vi "Nanonisframe.vi"(0 "x":dbl, 1 "z":dbl) -> (8 "X Out":dbl, 10 "Z Out":dbl, 11 "Target X":dbl, 12 "Speed":dbl, 13 "Target Z":dbl, 14 "FO X":dbl, 15 "FO Z":dbl, 16 "FW":dbl, 17 "FH":dbl)   [LabVIEW 2017]
uses:
  <userlib>/Nanonis Prog Interface V5/Nanonis Prog Interface.lvlib
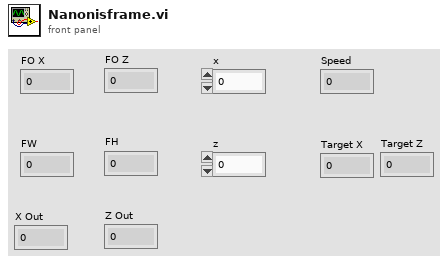
[diagram p1: front panel]
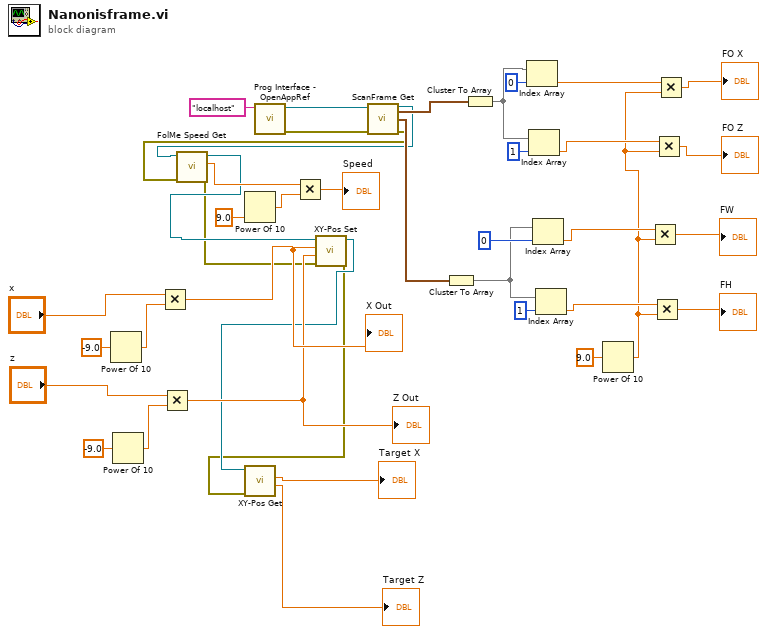
[diagram p0: block diagram]
diagram:
  n1 = Power Of 10(x=-9.0) -> (10^x=w16:dbl)
  n2 = Power Of 10(x=-9.0) -> (10^x=w13:dbl)
  n3 = Multiply(x="x", y=w16) -> (x*y=w9:dbl)
  "X Out" <- w9
  n4 = Multiply(x="z", y=w13) -> (x*y=w8:dbl)
  "Z Out" <- w8
  n5 = Power Of 10(x=9.0) -> (10^x=w19:dbl)
  n6 = call <userlib>:"Prog Interface - OpenAppRef.vi"("Machine name (local machine IP)"="localhost") -> ("Error out"=w4:errorcluster, "Application reference"=w40:refnum<vi>)  [unwired: 5 in]
  n7 = call <userlib>:"ScanFrame Get.vi"("Application ref in"=w40, "error in (no error)"=w4) -> ("Application ref out"=w21:refnum<vi>, "Center coordinates (m)"=w39:cluster{"Xc":sgl, "Yc":sgl}, "Size (m)"=w35:cluster{"Width":sgl, "Height":sgl}, "error out"=w3:errorcluster)  [unwired: 9 in, 1 out]
  n8 = call <userlib>:"FolMe Speed Get.vi"("error in (no error)"=w3, "Application ref in"=w21) -> ("error out"=w2:errorcluster, "Speed (m/s)"=w18:sgl, "Application ref out"=w10:refnum<vi>)  [unwired: 4 in, 1 out]
  n9 = Multiply(x=w18, y=w19) -> (x*y=→"Speed":dbl)
  n10 = call <userlib>:"XY-Pos Set.vi"("error in (no error)"=w2, "Y (m)"=w8, "X (m)"=w9, "Application ref in"=w10) -> ("error out"=w1:errorcluster, "Application ref out"=w7:refnum<vi>)  [unwired: 4 in]
  n11 = call <userlib>:"XY-Pos Get.vi"("error in (no error)"=w1, "Application ref in"=w7) -> ("Y (m)"=→"Target Z":sgl, "X (m)"=→"Target X":sgl)  [unwired: 5 in, 2 out]
  n12 = Cluster To Array(cluster=w35) -> (array=w32:sgl[])
  n13 = Cluster To Array(cluster=w39) -> (array=w38:sgl[])
  n14 = Index Array(array=w38, index=0) -> (element=w31:sgl)
  n15 = Index Array(array=w38, index=1) -> (element=w30:sgl)
  n16 = Index Array(array=w32, index=0) -> (element=w29:sgl)
  n17 = Index Array(array=w32, index=1) -> (element=w28:sgl)
  n18 = Power Of 10(x=9.0) -> (10^x=w26:dbl)
  n19 = Multiply(x=w29, y=w26) -> (x*y=→"FW":dbl)
  n20 = Multiply(x=w28, y=w26) -> (x*y=→"FH":dbl)
  n21 = Multiply(x=w30, y=w26) -> (x*y=→"FO Z":dbl)
  n22 = Multiply(x=w31, y=w26) -> (x*y=→"FO X":dbl)
